vi "VMR API Class.vi"() -> ()   [LabVIEW 2020]
uses:
  VoiceMeeterRemote/VoiceMeeterRemote/VoiceMeeterRemote.lvclass
panel:
  in  "VMR API":refnum<class "VoiceMeeterRemote.lvclass">
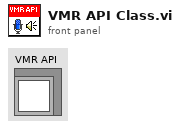
[diagram p1: front panel]
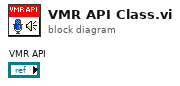
[diagram p0: block diagram]
diagram:
